vi "download_device_list.vi"(9 "port":u16, 10 "host":string, 11 "path in":path=path "hl2ss_ulm.dll") -> (0 "size":u64, 1 "port":u16, 2 "host":string, 3 "path out":path, 4 "query":u64, 5 "device_list_handle":u64)   [LabVIEW 2023]
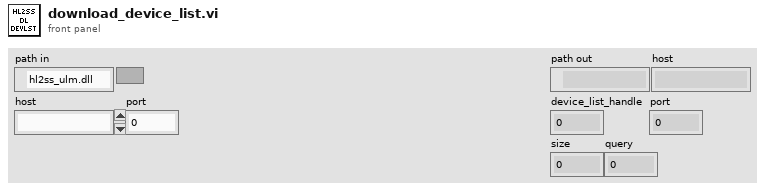
[diagram p1: front panel]
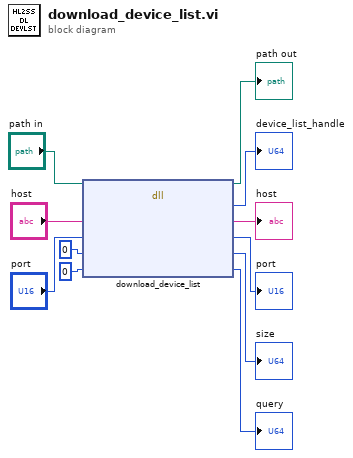
[diagram p0: block diagram]
diagram:
  n1 = dll-call lib="C:/Users/jcds/Documents/GitHub/hl2ss/extensions/client_labview/hl2ss_ulm.dll" fn="download_device_list"(path in="path in", "host"="host", "port"="port", "size"=u64 0, "query"=u64 0) -> (path out=→"path out":path, "return type"=→"device_list_handle":u64, "host"=→"host":string, "port"=→"port":u16, "size"=→"size":u64, "query"=→"query":u64)  [unwired: 2 in, 1 out]
